vi "ZenPlusOP300_refaire.vi"(1 "image":string, 5 "Refaire":T1=enum."Scan", 6 "Pédale":bool, 7 "Cas ok":T1=enum."Scan", 8 "errin":errorcluster, 9 "test ok ?":bool, 10 "MSG Jerome":string, 11 "Visa Pedale":refnum<visa-resource-name>) -> (0 "errout":errorcluster, 3 "Next":T1=enum."Scan")   [LabVIEW 2020]
uses:
  OP600ZP_state.ctl
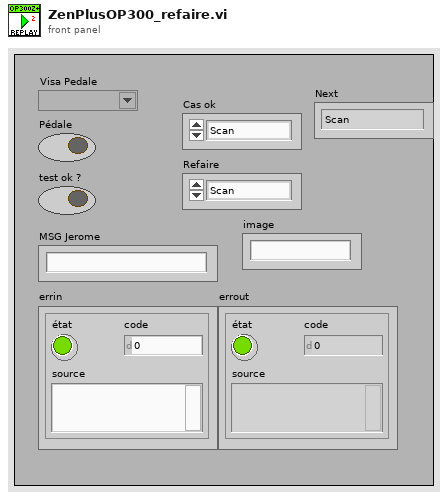
[diagram p1: front panel]
types:
  T1 = typedef "OP600ZP_state.ctl" = enum16{"Null", "Demarrage", "Init", "Scan", "Sealing", "VAT", "Iso", "Conti", "CAN Resistance", "Softs", "MCU", "OCV", "DTC", "PreCharge", "PackVoltage", "Capacitance", "Current + DCIR", "DataDyn", "Crash", "Next", "Comext"}
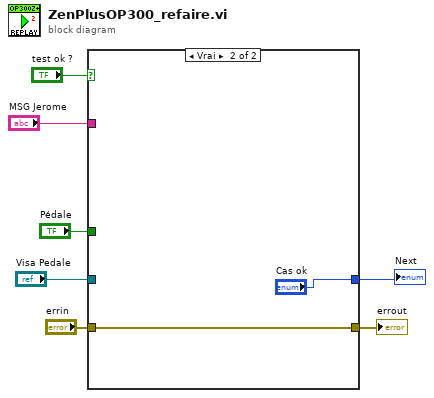
[diagram p0: block diagram]
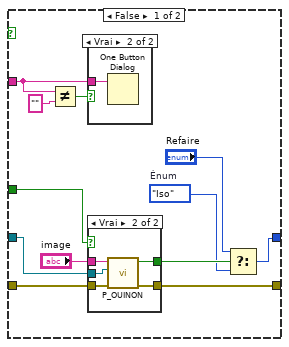
[diagram p2: hidden frame]
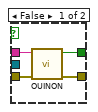
[diagram p4: hidden frame]
diagram:
  n1 = case shown="Vrai" "test ok ?" {
    tunnel: "errin" -> [w19 w31]
    tunnel: [w18 w31] -> w7
    tunnel: "Visa Pedale" -> [w17 _]
    tunnel: "MSG Jerome" -> [w13 _]
    tunnel: "Pédale" -> [w16 _]
    tunnel: [w10 "Cas ok"] -> w1
    frame False {
      w9 = OP600ZP_state."Iso"  # Énum
      n2 = Not Equal?(x=w13, y="") -> (x != y?=w11:bool)
      n3 = case shown="Vrai" w11 {
        tunnel: w13 -> [_ w20]
        frame False {
        }
        frame True {
          n4 = One Button Dialog(message=w20) -> ()  [unwired: 1 in, 1 out]
        }
      }
      n5 = case shown="Vrai" w16 {
        tunnel: "image" -> [w21 w29]
        tunnel: w19 -> [w24 w28]
        tunnel: [w23 w27] -> w18
        tunnel: [w22 w26] -> w14
        tunnel: w17 -> [_ w25]
        frame False {
          n6 = call "OUINON.vi"("errin"=w24, "image"=w21) -> ("error out"=w23:errorcluster, "OUI/NON"=w22:bool)  [unwired: 8 in]
        }
        frame True {
          n7 = call "P_OUINON.vi"("errin"=w28, "VISAin"=w25, "Image"=w29) -> ("error out"=w27:errorcluster, "=OUI?"=w26:bool)  [unwired: 7 in]
        }
      }
      n8 = Select(t="Refaire", s=w14, f=w9) -> (s? t:f=w10:T1)
    }
    frame True {
    }
  }
  "errout" <- w7
  "Next" <- w1
